vi "Test - My Singleton Module - Do Something 1.vi"(8 "error in (no error)":errorcluster) -> (0 "error out":errorcluster, 3 "Pass":bool)   [LabVIEW 2023]
doc: "_____\nCreated using DQMH Event Scripter 6.1.0.128."
uses:
  Libraries/My Singleton Module/My Singleton Module.lvlib
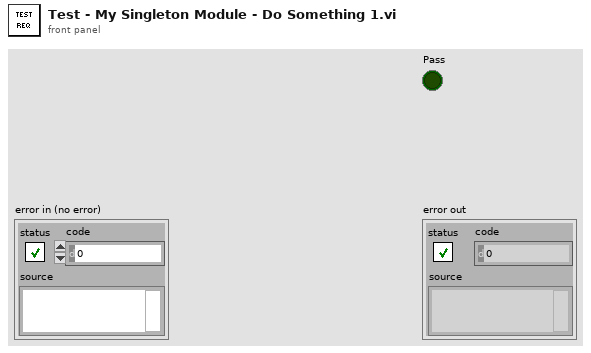
[diagram p1: front panel]
types:
  T1 = typedef "My Singleton Module.lvlib/Broadcast Events--cluster.ctl" = cluster{"Module Did Init":refnum<user-event>, "Status Updated":refnum<user-event>, "Error Reported":refnum<user-event>, "Did Something":refnum<user-event>, "Module Did Stop":refnum<user-event>, "Update Module Execution Status":refnum<user-event>}
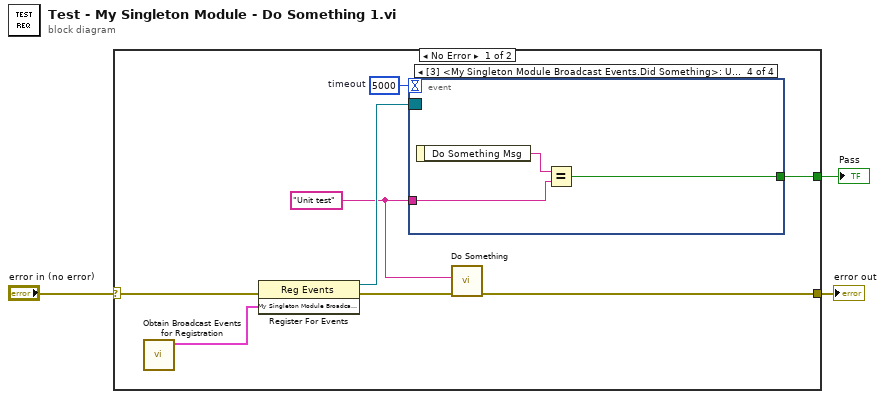
[diagram p0: block diagram]
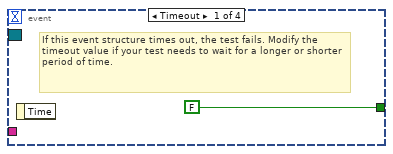
[diagram p2: hidden frame]
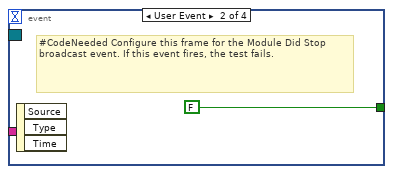
[diagram p3: hidden frame]
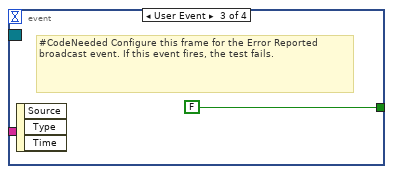
[diagram p4: hidden frame]
diagram:
  n1 = case shown="No Error" "error in (no error)" {
    selector: "error in (no error)" -> [w11 w18]
    tunnel: [w10 w18] -> w2
    tunnel: [w5 _] -> w1
    frame No Error {
      w4 = "Unit test" ("Do Something Message")
      w6 = 5000  # timeout
      n2 = call "Obtain Broadcast Events for Registration.vi"() -> ("My Singleton Module Broadcast Events"=w8:T1)  [unwired: 9 in, 2 out]
      n3 = register-events(error in=w11, w8) -> (reference out=w7:refnum<event-registration>, error out=w9:errorcluster)  [unwired: 1 in]
      n4 = event shown="[3] <My Singleton Module Broadcast Events.Did Something>: User Event" {
        selector: w7 -> [_ _ _ _]
        dyn-events: _ -> [_ _ _ _]
        timeout: w6 -> [_ _ _ _]
        tunnel: [FALSE FALSE FALSE w15] -> w5
        tunnel: w4 -> [_ _ _ w16]
        event Timeout {
          # "If this event structure times out, the test fails. Modify the timeout value if your test needs to wait for a longer or shorter period of time."
          n5 = event-data() -> ()  [unwired: 1 in, 1 out]
        }
        event User Event {
          # "#CodeNeeded Configure this frame for the Module Did Stop broadcast event. If this event fires, the test fails."
          n6 = event-data() -> ()  [unwired: 1 in, 3 out]
        }
        event User Event {
          # "#CodeNeeded Configure this frame for the Error Reported broadcast event. If this event fires, the test fails."
          n7 = event-data() -> ()  [unwired: 1 in, 3 out]
        }
        event User Event {
          n8 = event-data() -> ("Do Something Msg"=w17:string)  [unwired: 1 in]
          n9 = Equal?(x=w17, y=w16) -> (x = y?=w15:bool)
        }
      }
      n10 = call "Do Something.vi"("error in (no error)"=w9, "Do Something Message"=w4) -> ("error out"=w10:errorcluster)  [unwired: 9 in]
    }
    frame Error {
    }
  }
  "error out" <- w2
  "Pass" <- w1
